vi "Set Tree custom symbols.vi"(8 "error in":errorcluster, 9 "HSE Project?":bool, 10 "Project Name":string, 11 "TreeControl in":refnum<vi>) -> (0 "error out":errorcluster, 2 "Map":map{T1, i32}(c390), 3 "TreeControl out":refnum<vi>)   [LabVIEW 2020, in "Panther Dashboard.lvlib"]
uses:
  Panther Dashboard.lvlib
  Glyphs--enum.ctl
  <vilib>/Utility/Data Type/NI_Data Type.lvlib
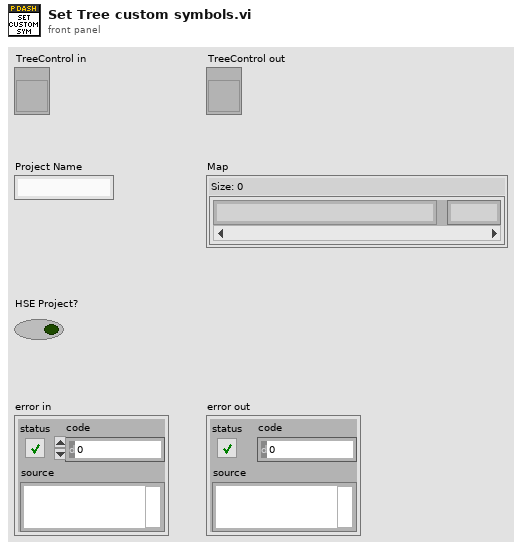
[diagram p1: front panel]
types:
  T1 = typedef "Panther Dashboard.lvlib/Glyphs--enum.ctl" = enum16{"Singleton", "SingletonRun", "SingletonDepencencies", "SingletonDependenciesRun", "Cloneable", "CloneableRun", "CloneableDependencies", "CloneableDependenciesRun", "HSE_Singleton", "HSE_SingletonRun", "HSE_SingletonDependencies", "HSE_SingletonDependenciesRun", "HSE_Cloneable", "HSE_CloneableRun", "HSE_CloneableDependencies", "HSE_CloneableDependenciesRun", "DQMH_Proj", "HSE_Proj", "Bad"}
  T2 = typedef "imagedata.ctl" = cluster{"image type":i32, "image depth":i32, "image":u8[], "mask":u8[], "colors":u32[], "Rectangle":cluster{"left":i16, "top":i16, "right":i16, "bottom":i16}}
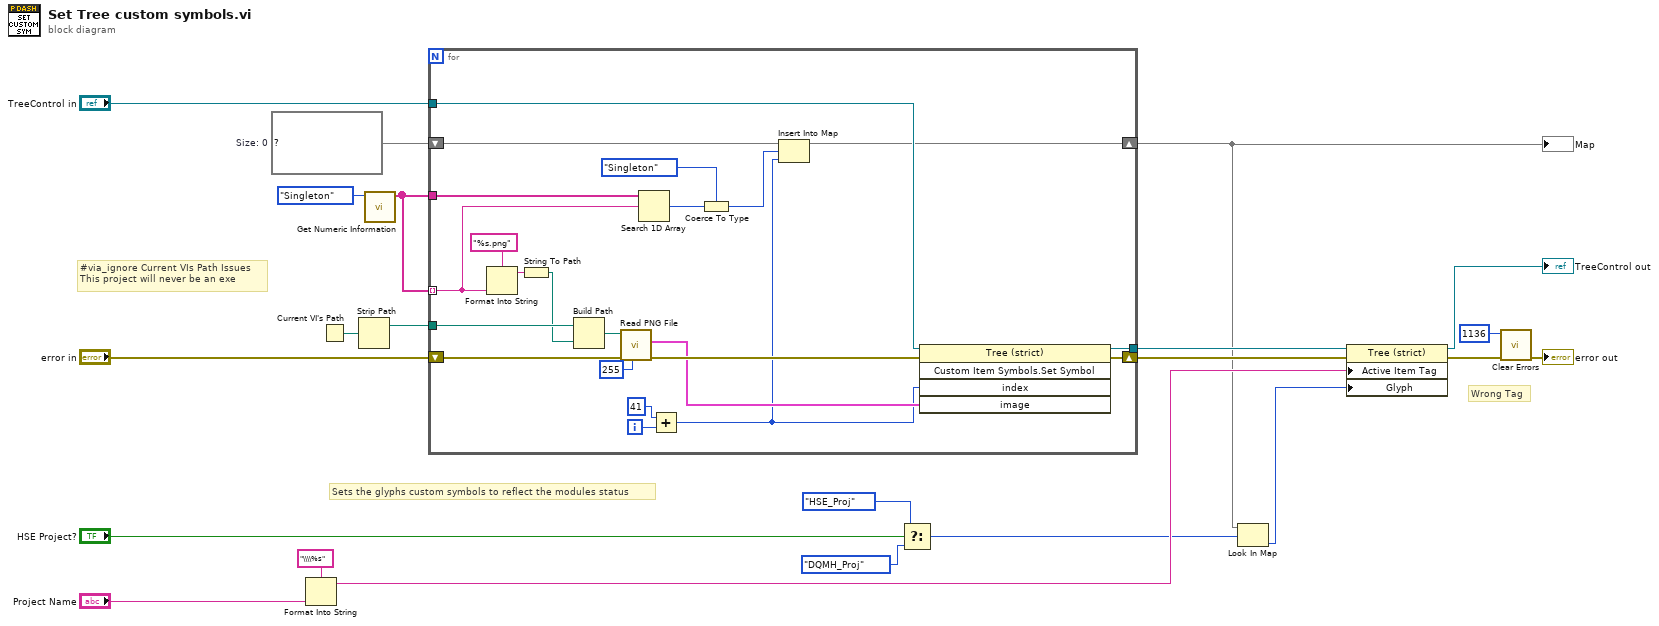
[diagram p0: block diagram]
diagram:
  w7 = map{T1, i32} {}  # Size: 0
  # "Wrong Tag"
  # "#via_ignore Current VIs Path Issues\nThis project will never be an exe"
  # "Sets the glyphs custom symbols to reflect the modules status"
  n1 = Format Into String(format string="\\\\%s", "Project Name") -> (resulting string=w13:string)  [unwired: 2 in, 1 out]
  n2 = Current VI's Path() -> (path=w15:path)
  n3 = Strip Path(path=w15) -> (stripped path=w14:path)  [unwired: 1 out]
  n4 = call <vilib>:"Get Numeric Information.vi"("variant"=Glyphs--enum."Singleton") -> ("enum names"=w8:string[])  [unwired: 7 in, 3 out]
  n5 = for {
    tunnel: w14 -> [w41]
    tunnel: "TreeControl in" -> [w37]
    tunnel: [w36] -> w11
    shift-right: [w43] -> w20
    shift-left: "error in" -> [w42]
    tunnel: w8 -> [w28] mode=indexing
    tunnel: w8 -> [w32]
    shift-right: [w30] -> w6
    shift-left: w7 -> [w31]
    i -> [w39]
    n6 = Format Into String(format string="%s.png", w28) -> (resulting string=w34:string)  [unwired: 2 in, 1 out]
    n7 = String To Path(string=w34) -> (path=w23:path)
    n8 = Build Path(base path=w41, name or relative path=w23) -> (appended path=w24:path)
    n9 = call <vilib>:"Read PNG File.vi"("Transparency Thresh"=u8 255, "error in (no error)"=w42, "path to PNG file"=w24) -> ("error out"=w44:errorcluster, "image data"=w38:T2)  [unwired: 6 in, 1 out]
    n10 = Search 1D Array(1D array=w32, element=w28) -> (index of element=w27:i32)  [unwired: 1 in]
    n11 = Add(x=41 ("Index"), y=w39) -> (x+y=w29:i32)
    n12 = Coerce To Type(0:w27, 1:Glyphs--enum."Singleton") -> (2:w25:T1)
    n13 = Insert Into Map(map in=w31, key=w25, value=w29) -> (map out=w30:map{T1, i32})  [unwired: 2 out]
    n14 = invoke on="Invoke Node" class="Tree (strict)" method="Custom Item Symbols.Set Symbol"(reference=w37, error in=w44, "index"=w29, "image"=w38) -> (reference out=w36:refnum<vi>, error out=w43:errorcluster)  [unwired: 1 in, 3 out]
  }
  "Map" <- w6
  n15 = Select(t=Glyphs--enum."HSE_Proj", s="HSE Project?", f=Glyphs--enum."DQMH_Proj") -> (s? t:f=w2:T1)
  n16 = Look In Map(map=w6, key=w2) -> (value=w1:i32)  [unwired: 1 in, 1 out]
  n17 = property class="Tree (strict)"(reference=w11, error in=w20, "Active Item Tag"=w13, "Glyph"=w1) -> (reference out=→"TreeControl out":refnum<vi>, error out=w21:errorcluster)
  n18 = call <vilib>:"Clear Errors.vi"("error in (no error)"=w21, "specific error code to clear (0: all)"=1136) -> ("error out"=→"error out":errorcluster)  [unwired: 4 in, 1 out]
